vi "GetAllTriangles.vi"() -> (3 "AllTriangles":T1[](array[typedef]))   [LabVIEW 2014]
uses:
  TypeDefs/TriangleFace.ctl
  TypeDefs/Point3D.ctl
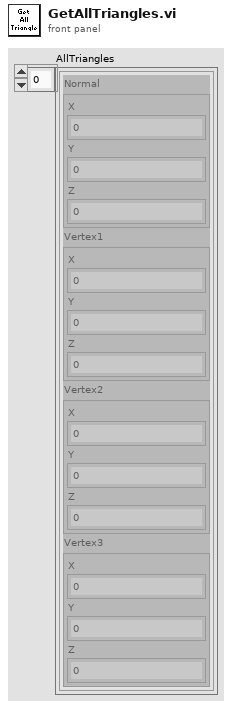
[diagram p1: front panel]
types:
  T1 = typedef "TriangleFace.ctl" = cluster{"Normal":T2, "Vertex1":T2, "Vertex2":T2, "Vertex3":T2}
  T2 = typedef "Point3D.ctl" = cluster{"X":sgl, "Y":sgl, "Z":sgl}
  T3 = enum16{"Add", "Get", "Scale", "Rotate", "Translate", "Symmetry"}
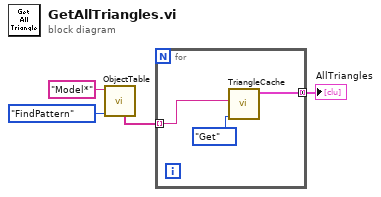
[diagram p0: block diagram]
diagram:
  n1 = call "ObjectTable.vi"("ObjectStoreSelector"=enum16{"New", "Find", "FindPattern", "GetTable"}."FindPattern", "Name"="Model*") -> ("Names"=w2:string[])  [unwired: 5 in, 4 out]
  n2 = for {
    tunnel: w2 -> [w6] mode=indexing
    tunnel: [w5] -> w1 mode=concatenating
    n3 = call "TriangleCache.vi"("TriangleOperations"=T3."Get", "ModelName"=w6) -> ("TrianglesOut"=w5:T1[])  [unwired: 9 in]
  }
  "AllTriangles" <- w1
